vi "Write Warming Done Value.vi"(8 "error in (no error)":errorcluster, 10 "Value":bool, 11 "Generic Card in":refnum<class "Generic Card.lvclass">) -> (0 "error out":errorcluster, 3 "Generic Card out":refnum<class "Generic Card.lvclass">)   [LabVIEW 2014, in "Generic Instrument.lvlib" / "Generic Card.lvclass"]
uses:
  Generic Card.lvclass
  Generic Card.lvclass/Generic Card.ctl
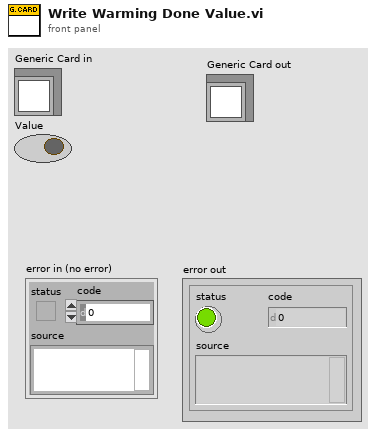
[diagram p1: front panel]
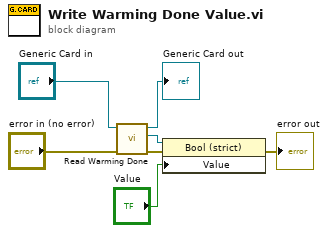
[diagram p0: block diagram]
diagram:
  n1 = call "Read Warming Done.vi"("error in (no error)"="error in (no error)", "Generic Card in"="Generic Card in") -> ("error out"=w6:errorcluster, "Warming Done"=w7:refnum<vi>, "Generic Card out"=→"Generic Card out":refnum<class "Generic Card.lvclass">)  [unwired: 7 in]
  n2 = property class="Bool (strict)"(reference=w7, error in=w6, "Value"="Value") -> (error out=→"error out":errorcluster)  [unwired: 1 out]
